vi "Pfeiffer-RVC300.set mode.vi"(0 "i ref in":refnum<vi>, 1 "regulationMode":T1, 3 "ms timeout (10000)":i32=10000, 5 "error in (no error)":errorcluster) -> (14 "i ref out":refnum<vi>, 17 "timed out":bool, 19 "error out":errorcluster)   [LabVIEW 2014, in "Pfeiffer-RVC300.lvlib"]
doc: "Sets the mode to pressure regulation, flow regulation or wait.\n\nLicense Agreement for this software:\n\nCopyright (C)\nMax-Planck-Institut für Kernphysik\nSaupfercheckweg 1\n69117 Heidelberg\nGermany\n\nContact: christopher.borgmann@mpi-hd.mpg.de\n\nThis program is free software: you can redistribute it and/or modify \nit under the terms of the GNU General Public License as published by\nthe Free Software Foundation, either version 3 of the License, or\n(at your option) any later version.\n\nThis program is distributed in the hope that it will be useful,\nbut WITHOUT ANY WARRANTY; without even the implied warranty of\nMERCHANTABILITY or FITNESS FOR A PARTICULAR PURPOSE. See the\nGNU General Public License for more details.\n\nYou should have received a copy of the GNU General Public License\nalong with this program. If not, see <http://www.gnu.org/licenses/>.\n\nMax-Planck-Institut für Kernphysik\nSaupfercheckweg 1, 69117 Heidelberg, Germany\nFor all questions and ideas contact: christopher.borgmann@mpi-hd.mpg.de\nLast update: 08.07.2010"
uses:
  Pfeiffer-RVC300.lvlib
  CSCore/CSApplicationBaseClasses/DeviceBase/DeviceBase.lvlib
  CSlibraries-extern/DimLVEvent/LVDimInterface/LVDimInterface.lvlib
  Pfeiffer-RVC300.regulation mode.ctl
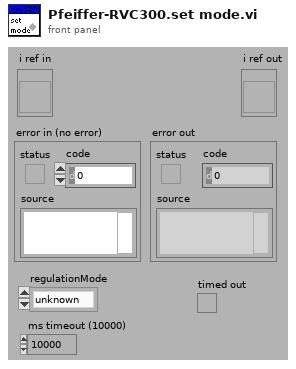
[diagram p1: front panel]
types:
  T1 = typedef "Pfeiffer-RVC300.lvlib/Pfeiffer-RVC300.regulation mode.ctl" = enum16{"unknown", "Pressure", "Flow", "Wait"}
  T2 = typedef "Pfeiffer-RVC300.lvlib/Pfeiffer-RVC300.i attribute.ctl" = cluster{"interfaceInitialized":bool, "VISAResource":refnum<visa-resource-name>, "WaitingTime":u32, "nomValues":T3, "actValues":T3}
  T3 = typedef "Pfeiffer-RVC300.lvlib/Pfeiffer-RVC300.parameters.ctl" = cluster{"regulationMode":T1, "valveType":string, "sensorType":string, "valveState":string, "flow":dbl, "pressure":dbl, "serviceIDs":cluster{"regulationModeID":i32, "valveTypeID":i32, "sensorTypeID":i32, "valveStateID":i32, "flowID":i32, "pressureID":i32}}
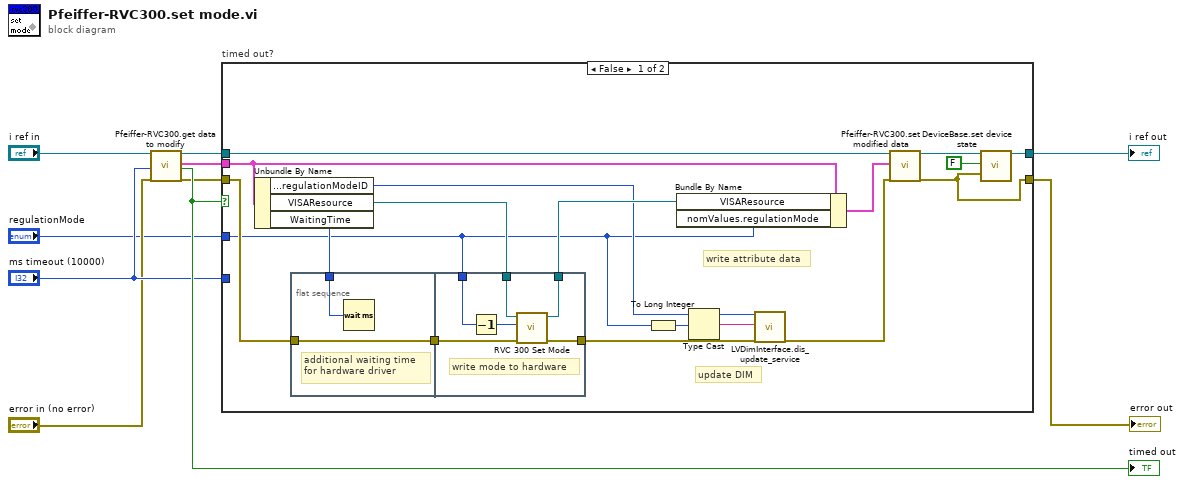
[diagram p0: block diagram]
diagram:
  n1 = call "Pfeiffer-RVC300.get data to modify.vi"("i ref in"="i ref in", "ms timeout (10000)"="ms timeout (10000)", "error in (no error)"="error in (no error)") -> ("i ref out"=w4:refnum<vi>, "i attribute"=w2:T2, "timed out"=w7:bool, "error out"=w3:errorcluster)  [unwired: 13 in]
  "timed out" <- w7
  n2 = case "timed out?" shown="False" w7 {
    tunnel: [w25 w38] -> w9
    tunnel: w4 -> [w28 w38]
    tunnel: [w23 w37] -> w8
    tunnel: w3 -> [w22 w37]
    tunnel: w2 -> [w20 _]
    tunnel: "ms timeout (10000)" -> [_ _]
    tunnel: "regulationMode" -> [w15 _]
    frame False {
      # "write attribute data"
      # "update DIM"
      n3 = Unbundle By Name(w20) -> ("nomValues.serviceIDs.regulationModeID"=w16:i32, "VISAResource"=w18:refnum<visa-resource-name>, "WaitingTime"=w17:u32)
      n4 = flat-sequence {
        tunnel: w22 -> [w30]
        tunnel: [w30] -> w21
        tunnel: w17 -> [w29]
        tunnel: w21 -> [w36]
        tunnel: w18 -> [w35]
        tunnel: w15 -> [w34]
        tunnel: [w33] -> w12
        tunnel: [w32] -> w19
        frame #0 {
          # "additional waiting time \nfor hardware driver"
          n5 = Wait (ms)(milliseconds to wait=w29) -> ()  [unwired: 1 out]
        }
        frame #1 {
          # "write mode to hardware"
          n6 = Decrement(x=w34) -> (x-1=w31:T1)
          n7 = call "RVC 300 Set Mode.vi"("error in"=w36, "Mode"=w31, "Resource Name"=w35) -> ("error out"=w33:errorcluster, "Resource Name out"=w32:refnum<visa-resource-name>)  [unwired: 3 in]
        }
      }
      n8 = To Long Integer(number=w15) -> (32bit integer=w11:i32)
      n9 = Bundle By Name(cluster=w20, "VISAResource"=w19, "nomValues.regulationMode"=w15) -> (w27:T2)
      n10 = Type Cast(x=w11) -> (*(type *) &x=w14:string)  [unwired: 1 in]
      n11 = call "LVDimInterface.dis_update_service.vi"("my_serviceID"=w16, "data"=w14, "error in (no error)"=w12) -> ("error out"=w13:errorcluster)  [unwired: 14 in, 2 out]
      n12 = call "Pfeiffer-RVC300.set modified data.vi"("i ref in"=w28, "i attribute"=w27, "error in (no error)"=w13) -> ("i ref out"=w26:refnum<vi>, "error out"=w23:errorcluster)  [unwired: 15 in]
      n13 = call "DeviceBase.set device state.vi"("i ref in"=w26, "implicit"=FALSE, "device error"=w23) -> ("i ref out"=w25:refnum<vi>)  [unwired: 14 in, 2 out]
    }
    frame True {
    }
  }
  "error out" <- w8
  "i ref out" <- w9
